vi "xPCGetParamIdx.vi"(3 "error in (no error)":errorcluster, 4 "blockpath":string, 5 "parametername":string, 6 "port":i32) -> (0 "error out":errorcluster, 1 "identifier":i32, 2 "port copy":i32)   [LabVIEW 2018]
uses:
  XPCAPI.DLL
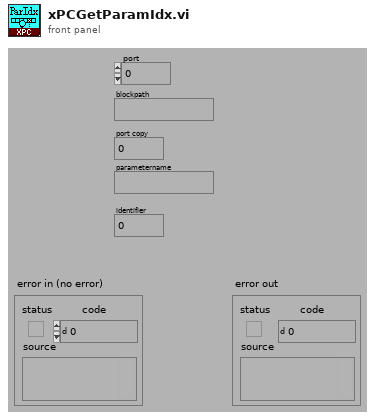
[diagram p1: front panel]
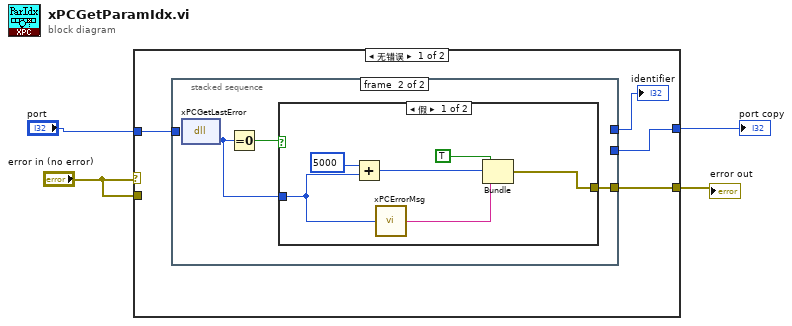
[diagram p0: block diagram]
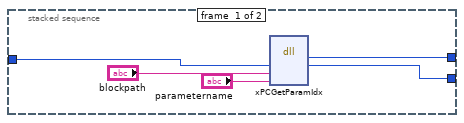
[diagram p2: hidden frame]
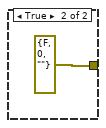
[diagram p3: hidden frame]
diagram:
  n1 = case shown="无错误" "error in (no error)" {
    tunnel: [w8 w25] -> w4
    tunnel: "error in (no error)" -> [_ w25]
    tunnel: "port" -> [w6 w24]
    tunnel: [w7 w24] -> w2
    frame No Error {
      n2 = stacked-sequence {
        tunnel: [w10 _] -> w7
        tunnel: [_ w14] -> w8
        tunnel: w6 -> [w11 _]
        tunnel: [w9 _] -> w5
        frame #0 {
          n3 = dll-call lib="PTH2Dabs CUsers19320Desktop上下位机联机测试\nxpcapi.dll" fn="xPCGetParamIdx"("port"=w11, "blockpath"="blockpath", "parametername"="parametername") -> (w9:i32, "port"=w10:i32)  [unwired: 5 in, 2 out]
        }
        frame #1 {
          n4 = dll-call lib="PTH2Dabs CUsers19320Desktop上下位机联机测试\nxpcapi.dll" fn="xPCGetLastError"() -> (w15:i32)  [unwired: 3 in, 2 out]
          n5 = Equal To 0?(x=w15) -> (x = 0?=w16:bool)
          n6 = case shown="假" w16 {
            tunnel: w15 -> [w18 _]
            tunnel: [w19 errorcluster {"status"=FALSE, "code"=0, "source"=""} ("error out")] -> w14
            frame False {
              n7 = Add(x=5000 ("y"), y=w18) -> (x+y=w21:i32)
              n8 = call "xPCErrorMsg.vi"("error number"=w18) -> ("ErrorMsg"=w20:string)
              n9 = Bundle(TRUE, w21, "ErrorMsg"=w20) -> (w19:cluster{bool, i32, "ErrorMsg":string})  [unwired: 1 in]
            }
            frame True {
            }
          }
        }
      }
      "identifier" <- w5
    }
    frame Error {
    }
  }
  "port copy" <- w2
  "error out" <- w4
